vi "sub_LidarCluster.vi"(8 "Box Offset":dbl, 9 "군집원소 최소 갯수(threshold)":i32=80, 10 "군집원소 간 거리(threshold)":dbl=0.09 format="%#_13g", 11 "XY DATA":cluster{"X":dbl, "Y":dbl}[](array[cluster])) -> (1 "Box Point Array":cluster{dbl[], dbl[]}[](array[cluster]), 2 "Safe Box Plotting":cluster{dbl[], dbl[]}[](graph), 3 "Cluster Plotting":T1(graph))   [LabVIEW 2020]
panel:
  in  "탭 컨트롤":enum32{"인디케이터"}(tab)
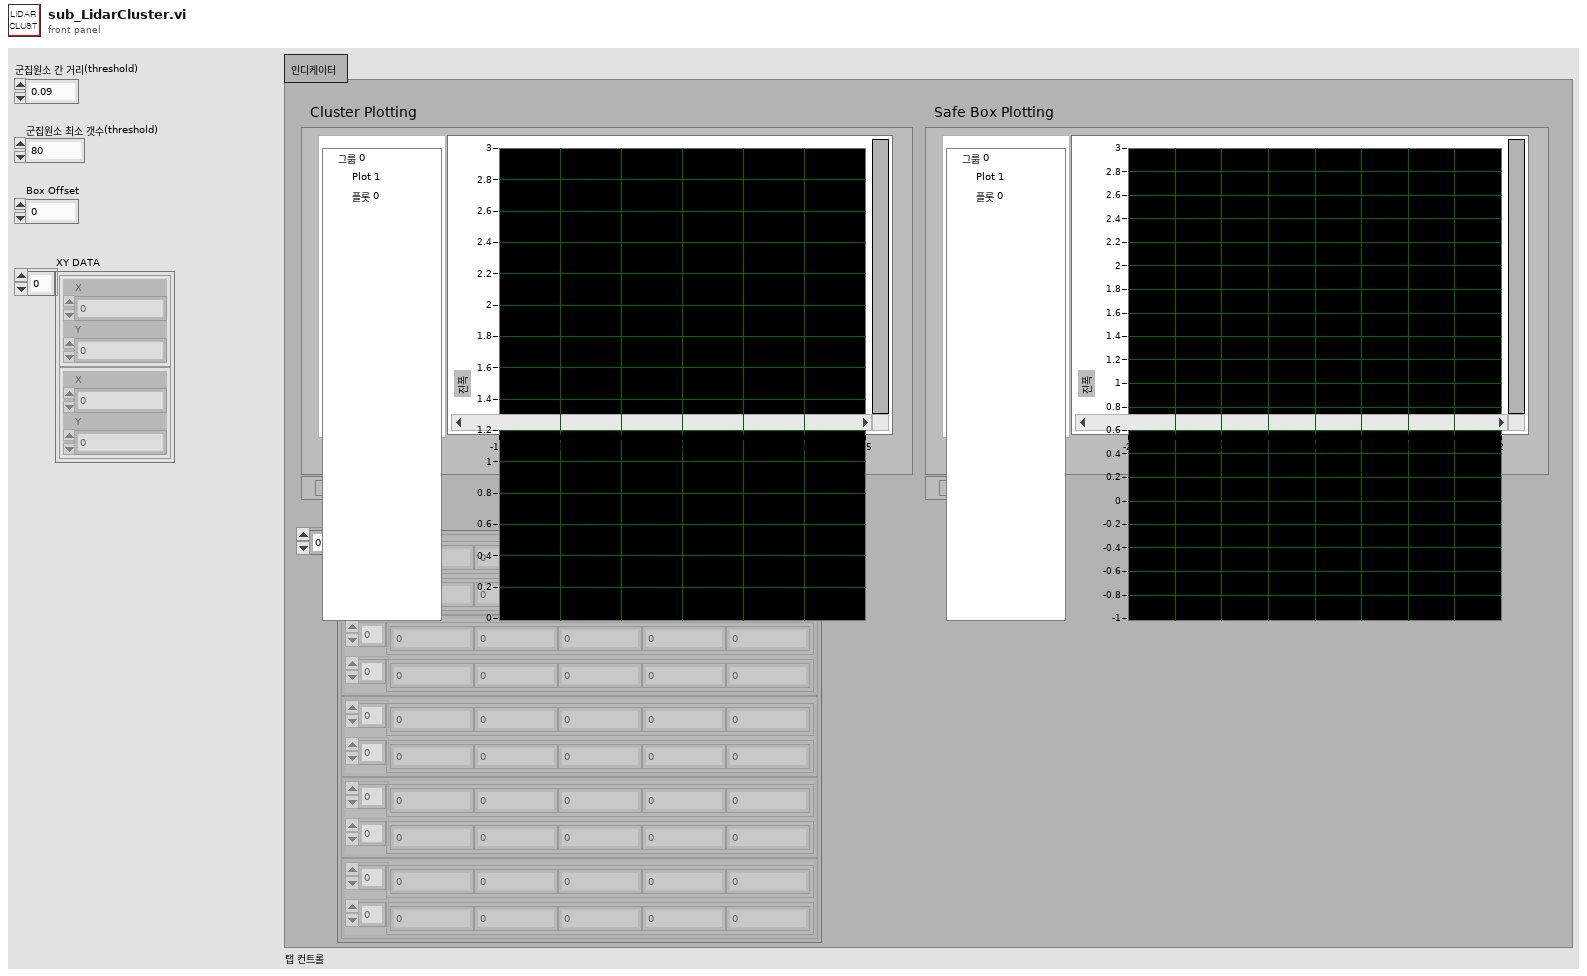
[diagram p1: front panel]
types:
  T1 = cluster{"최종 클러스터링 배열":cluster{"X":dbl, "Y":dbl}[]}[]
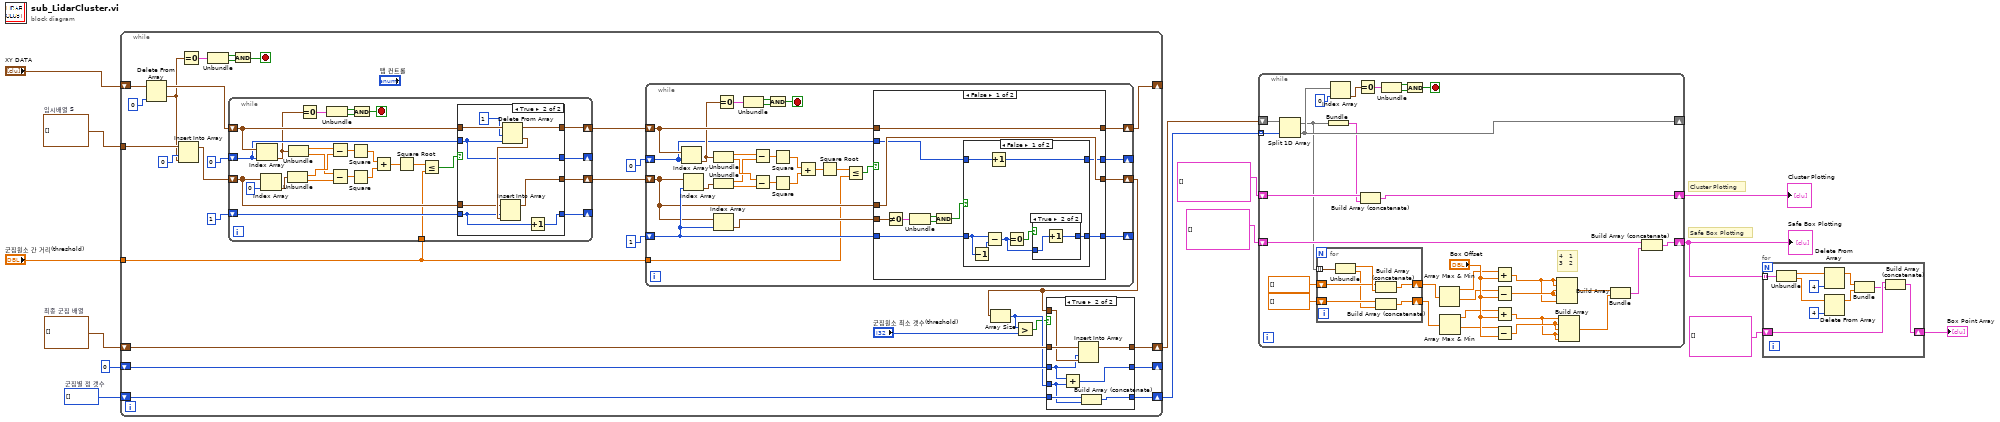
[diagram p0: block diagram]
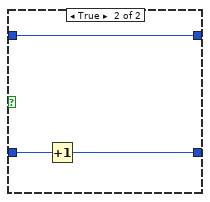
[diagram p3: hidden frame]
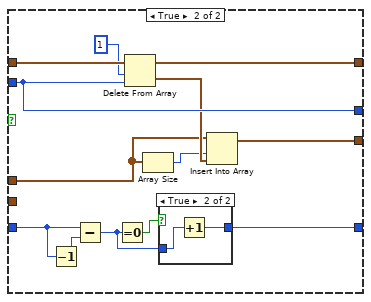
[diagram p4: hidden frame]
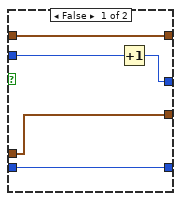
[diagram p6: hidden frame]
diagram:
  w6 = i32[] []  # 군집별 점 갯수
  w3 = cluster{"X":dbl, "Y":dbl}[] []  # 임시배열 S
  w4 = cluster{"X":dbl, "Y":dbl}[] []  # 최종 군집 배열
  # "Safe Box Plotting"
  # "Cluster Plotting"
  n1 = while {
    shift-right: [w36] -> _
    shift-left: "XY DATA" -> [w21]
    tunnel: w3 -> [w42]
    shift-right: [w30] -> w7
    shift-left: w4 -> [w34]
    shift-right: [w26] -> w9
    shift-left: w6 -> [w31]
    shift-right: [w27] -> _
    shift-left: 0 -> [w29]
    tunnel: "군집원소 간 거리(threshold)" -> [w15]
    stop <- w17 stop-if-true
    n2 = Delete From Array(array=w21, index=0 ("인덱스")) -> (deleted portion=w16:cluster{"X":dbl, "Y":dbl}, array with subset deleted=w32:cluster{"X":dbl, "Y":dbl}[])  [unwired: 1 in]
    n3 = Insert Into Array(array=w42, index=0 ("인덱스"), new element=w16) -> (w41:cluster{"X":dbl, "Y":dbl}[])
    n4 = Equal To 0?(x=w16) -> (x = 0?=w20:cluster{"X":bool, "Y":bool})
    n5 = Unbundle(w20) -> ("X"=w19:bool, "Y"=w18:bool)
    n6 = while {
      shift-right: [w119] -> w39
      shift-left: w41 -> [w121]
      shift-right: [w122] -> w38
      shift-left: w32 -> [w124]
      shift-right: [w120] -> _
      shift-left: 0 -> [w123]
      shift-right: [w117] -> _
      shift-left: 1 -> [w118]
      tunnel: w15 -> [w111]
      stop <- w113 stop-if-true
      n7 = Index Array(array=w124, index=w123) -> (element=w114:cluster{"X":dbl, "Y":dbl})
      n8 = Index Array(array=w121, index=0 ("인덱스")) -> (element=w131:cluster{"X":dbl, "Y":dbl})
      n9 = Unbundle(w131) -> ("X"=w129:dbl, "Y"=w127:dbl)
      n10 = Unbundle(w114) -> ("X"=w130:dbl, "Y"=w128:dbl)
      n11 = Equal To 0?(x=w114) -> (x = 0?=w116:cluster{"X":bool, "Y":bool})
      n12 = Unbundle(w116) -> ("X"=w115:bool, "Y"=w112:bool)
      n13 = Subtract(x=w130, y=w129) -> (x-y=w136:dbl)
      n14 = Subtract(x=w128, y=w127) -> (x-y=w133:dbl)
      n15 = Square(x=w136) -> (x^2=w134:dbl)
      n16 = Square(x=w133) -> (x^2=w132:dbl)
      n17 = And(x=w115, y=w112) -> (x .and. y?=w113:bool)
      n18 = Add(x=w134, y=w132) -> (x+y=w135:dbl)
      n19 = Square Root(x=w135) -> (sqrt(x)=w126:dbl)
      n20 = Less Or Equal?(x=w126, y=w111) -> (x <= y?=w125:bool)
      n21 = case shown="True" w125 {
        tunnel: w124 -> [w138 w151]
        tunnel: w123 -> [w142 w143]
        tunnel: [w138 w149] -> w122
        tunnel: w121 -> [w140 w147]
        tunnel: [w141 w143] -> w120
        tunnel: [w140 w146] -> w119
        tunnel: w118 -> [w139 w145]
        tunnel: [w139 w144] -> w117
        frame False {
          n22 = Increment(x=w142) -> (x+1=w141:i32)
        }
        frame True {
          n23 = Delete From Array(array=w151, length=1 ("길이"), index=w143) -> (deleted portion=w148:cluster{"X":dbl, "Y":dbl}[], array with subset deleted=w149:cluster{"X":dbl, "Y":dbl}[])
          n24 = Insert Into Array(array=w147, index=w145, new element=w148) -> (w146:cluster{"X":dbl, "Y":dbl}[])
          n25 = Increment(x=w145) -> (x+1=w144:i32)
        }
      }
    }
    n26 = And(x=w19, y=w18) -> (x .and. y?=w17:bool)
    n27 = while {
      shift-right: [w59] -> w25
      shift-left: w39 -> [w51]
      shift-right: [w58] -> _
      shift-left: 1 -> [w52]
      shift-right: [w55] -> w36
      shift-left: w38 -> [w56]
      shift-right: [w50] -> _
      shift-left: 0 -> [w45]
      tunnel: w15 -> [w44]
      stop <- w48 stop-if-true
      n28 = Index Array(array=w56, index=w45) -> (element=w47:cluster{"X":dbl, "Y":dbl})
      n29 = Index Array(array=w51, index=w52) -> (element=w70:cluster{"X":dbl, "Y":dbl})
      n30 = Unbundle(w47) -> ("X"=w63:dbl, "Y"=w62:dbl)
      n31 = Unbundle(w70) -> ("X"=w61:dbl, "Y"=w60:dbl)
      n32 = Index Array(array=w51, index=w52) -> (element=w49:cluster{"X":dbl, "Y":dbl})
      n33 = Equal To 0?(x=w47) -> (x = 0?=w54:cluster{"X":bool, "Y":bool})
      n34 = Unbundle(w54) -> ("X"=w53:bool, "Y"=w46:bool)
      n35 = Subtract(x=w63, y=w61) -> (x-y=w69:dbl)
      n36 = Subtract(x=w62, y=w60) -> (x-y=w66:dbl)
      n37 = And(x=w53, y=w46) -> (x .and. y?=w48:bool)
      n38 = Square(x=w69) -> (x^2=w67:dbl)
      n39 = Square(x=w66) -> (x^2=w65:dbl)
      n40 = Add(x=w67, y=w65) -> (x+y=w68:dbl)
      n41 = Square Root(x=w68) -> (sqrt(x)=w64:dbl)
      n42 = Less Or Equal?(x=w64, y=w44) -> (x <= y?=w57:bool)
      n43 = case shown="False" w57 {
        tunnel: w51 -> [w73 w102]
        tunnel: [w73 w107] -> w59
        tunnel: [w75 w96] -> w58
        tunnel: w52 -> [w76 w100]
        tunnel: w45 -> [w72 w104]
        tunnel: [w71 w104] -> w50
        tunnel: w56 -> [w81 w106]
        tunnel: [w81 w105] -> w55
        tunnel: w49 -> [w80 _]
        frame False {
          n44 = Not Equal To 0?(x=w80) -> (x != 0?=w79:cluster{"X":bool, "Y":bool})
          n45 = Unbundle(w79) -> ("X"=w78:bool, "Y"=w74:bool)
          n46 = And(x=w78, y=w74) -> (x .and. y?=w77:bool)
          n47 = case shown="False" w77 {
            tunnel: w76 -> [w83 w94]
            tunnel: [w82 w93] -> w75
            tunnel: w72 -> [w88 w92]
            tunnel: [w87 w92] -> w71
            frame False {
              n48 = Decrement(x=w83) -> (x-1=w86:i32)
              n49 = Subtract(x=w83, y=w86) -> (x-y=w84:i32)
              n50 = Increment(x=w88) -> (x+1=w87:i32)
              n51 = Equal To 0?(x=w84) -> (x = 0?=w85:bool)
              n52 = case shown="True" w85 {
                tunnel: w84 -> [w89 w90]
                tunnel: [w89 w91] -> w82
                frame False {
                }
                frame True {
                  n53 = Increment(x=w90) -> (x+1=w91:i32)
                }
              }
            }
            frame True {
              n54 = Increment(x=w94) -> (x+1=w93:i32)
            }
          }
        }
        frame True {
          n55 = Decrement(x=w100) -> (x-1=w99:i32)
          n56 = Subtract(x=w100, y=w99) -> (x-y=w97:i32)
          n57 = Equal To 0?(x=w97) -> (x = 0?=w98:bool)
          n58 = Delete From Array(array=w106, length=1 ("길이"), index=w104) -> (deleted portion=w103:cluster{"X":dbl, "Y":dbl}[], array with subset deleted=w105:cluster{"X":dbl, "Y":dbl}[])
          n59 = Array Size ("XY 쌍의 갯수")(array=w102) -> (size(s)=w101:i32)
          n60 = case shown="True" w98 {
            tunnel: w97 -> [w108 w109]
            tunnel: [w108 w110] -> w96
            frame False {
            }
            frame True {
              n61 = Increment(x=w109) -> (x+1=w110:i32)
            }
          }
          n62 = Insert Into Array(array=w102, index=w101, new element=w103) -> (w107:cluster{"X":dbl, "Y":dbl}[])
        }
      }
    }
    n63 = Array Size ("XY 쌍의 갯수")(array=w25) -> (size(s)=w28:i32)
    n64 = Greater?(x=w28, y="군집원소 최소 갯수(threshold)") -> (0:w22:bool)
    n65 = case shown="True" w22 {
      tunnel: w25 -> [_ w161]
      tunnel: w34 -> [w154 w162]
      tunnel: [w154 w160] -> w30
      tunnel: w31 -> [w152 w157]
      tunnel: w29 -> [w153 w159]
      tunnel: w28 -> [_ w156]
      tunnel: [w153 w158] -> w27
      tunnel: [w152 w155] -> w26
      frame False {
      }
      frame True {
        n66 = Add(x=w159, y=w156) -> (x+y=w158:i32)
        n67 = Insert Into Array(array=w162, index=w159, new element=w161) -> (w160:cluster{"X":dbl, "Y":dbl}[])
        n68 = Build Array (concatenate)(w157, w156) -> (w155:i32[])
      }
    }
  }
  n69 = while {
    shift-right: [w193] -> w11
    shift-left: T1 [] -> [w184]
    shift-right: [w186] -> _
    shift-left: w7 -> [w192]
    tunnel: w9 -> [w180] mode=indexing
    shift-right: [w176] -> w12
    shift-left: cluster{dbl[], dbl[]}[] [] -> [w177]
    stop <- w187 stop-if-true
    # "4   1\n3   2"
    n70 = Split 1D Array(array=w192, index=w180) -> (first subarray=w173:cluster{"X":dbl, "Y":dbl}[], second subarray=w186:cluster{"X":dbl, "Y":dbl}[])
    n71 = for {
      tunnel: w173 -> [w200] mode=indexing
      shift-right: [w197] -> w175
      shift-left: dbl[] [] -> [w198]
      shift-right: [w194] -> w174
      shift-left: dbl[] [] -> [w196]
      n72 = Unbundle(w200) -> ("X"=w199:dbl, "Y"=w195:dbl)
      n73 = Build Array (concatenate)(w198, w199) -> (w197:dbl[])
      n74 = Build Array (concatenate)(w196, w195) -> (w194:dbl[])
    }
    n75 = Bundle(w173) -> (w183:cluster{cluster{"X":dbl, "Y":dbl}[]})  [unwired: 1 in]
    n76 = Index Array(array=w186, index=0 ("인덱스")) -> (element=w191:cluster{"X":dbl, "Y":dbl})
    n77 = Equal To 0?(x=w191) -> (x = 0?=w190:cluster{"X":bool, "Y":bool})
    n78 = Build Array (concatenate)(w184, w183) -> (w193:T1)
    n79 = Unbundle(w190) -> ("X"=w189:bool, "Y"=w188:bool)
    n80 = And(x=w189, y=w188) -> (x .and. y?=w187:bool)
    n81 = Array Max & Min(array=w175) -> (max value=w171:dbl, min value=w169:dbl)  [unwired: 2 out]
    n82 = Array Max & Min(array=w174) -> (max value=w170:dbl, min value=w168:dbl)  [unwired: 2 out]
    n83 = Add(x=w171, y="Box Offset") -> (x+y=w166:dbl)
    n84 = Subtract(x=w169, y="Box Offset") -> (x-y=w167:dbl)
    n85 = Add(x=w170, y="Box Offset") -> (x+y=w164:dbl)
    n86 = Subtract(x=w168, y="Box Offset") -> (x-y=w165:dbl)
    n87 = Build Array(w166, w166, w167, w167, w166) -> (w179:dbl[])
    n88 = Build Array(w164, w165, w165, w164, w164) -> (w178:dbl[])
    n89 = Bundle(w179, w178) -> (w163:cluster{dbl[], dbl[]})  [unwired: 1 in]
    n90 = Build Array (concatenate)(w177, w163) -> (w176:cluster{dbl[], dbl[]}[])
  }
  "Cluster Plotting" <- w11
  "Safe Box Plotting" <- w12
  n91 = for {
    tunnel: w12 -> [w210] mode=indexing
    shift-right: [w202] -> w14
    shift-left: cluster{dbl[], dbl[]}[] [] -> [w203]
    n92 = Unbundle(w210) -> (w209:dbl[], w206:dbl[])
    n93 = Delete From Array(array=w209, index=4 ("인덱스")) -> (array with subset deleted=w205:dbl[])  [unwired: 1 in, 1 out]
    n94 = Delete From Array(array=w206, index=4 ("인덱스")) -> (array with subset deleted=w204:dbl[])  [unwired: 1 in, 1 out]
    n95 = Bundle(w205, w204) -> (w201:cluster{dbl[], dbl[]})  [unwired: 1 in]
    n96 = Build Array (concatenate)(w203, w201) -> (w202:cluster{dbl[], dbl[]}[])
  }
  "Box Point Array" <- w14
